vi "ScriptTerminals.vi"(4 "SubVI Refnum":refnum<vi>, 5 "Terms":T1[](array[typedef]), 6 "IS CORE CASE? (f)":bool, 7 "Diag Refnum":refnum<vi>, 9 "error in":errorcluster, 10 "Messages":u8[](array[numeric]), 11 "Name":string) -> ()   [LabVIEW 2012, in "CThread.lvlib"]
uses:
  CThread.lvlib
  <vilib>/XNodeSupport/XNodeTermIDPair.ctl
  <vilib>/XNodeSupport/XNodeTermRef.ctl
  <vilib>/XNodeSupport/XNodeString.ctl
  <vilib>/Utility/miscctls.llb/LVPointTypeDef.ctl
  CRef/CRef.lvlib
  <vilib>/XNodeSupport/NI_XNodeSupport.lvlib
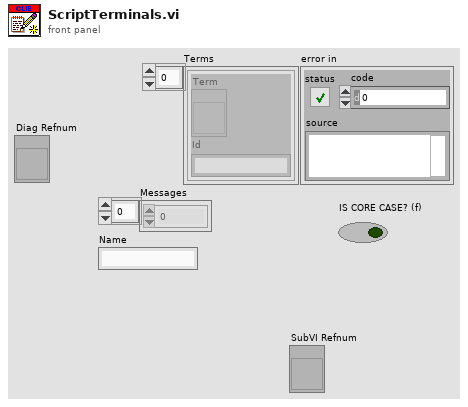
[diagram p1: front panel]
types:
  T1 = typedef "NI_XNodeSupport.lvlib/XNodeTermIDPair.ctl" = cluster{"Term":T2, "Id":T3}
  T2 = typedef "NI_XNodeSupport.lvlib/XNodeTermRef.ctl" = refnum<vi>
  T3 = typedef "NI_XNodeSupport.lvlib/XNodeString.ctl" = string
  T4 = typedef "LVPointTypeDef.ctl" = cluster{"Horizontal":i16, "Vertical":i16}
  T5 = enum16{"Create", "Get", "Set", "Static", "Release"}
  T6 = typedef "CRef.lvlib/Master Types.ctl" = enum8{"Null", "Boolean", "U8", "I8", "U16", "I16", "U32", "I32", "U64", "I64", "Single", "Double", "Extended", "CSG", "CDB", "CXT", "Boolean(Def)", "U8(Def)", "I8(Def)", "U16(Def)", "I16(Def)", "U32(Def)", "I32(Def)", "Reserved Def", "Reserved Def1", "Single(Def)", "Double(Def)", "Reserved Def2", "Reserved Def3", "Reserved Def4", "Reserved Def5", "Unsigned(Def)", "Signed(Def)", "Real(Def)", "Reserved Def6", "Numeric(Def)", "String"}
  T7 = typedef "LVRectTypeDef.ctl" = cluster{"Left":i16, "Top":i16, "Right":i16, "Bottom":i16}
  T8 = cluster{"Left":bool, "Top":bool, "Right":bool, "Bottom":bool}
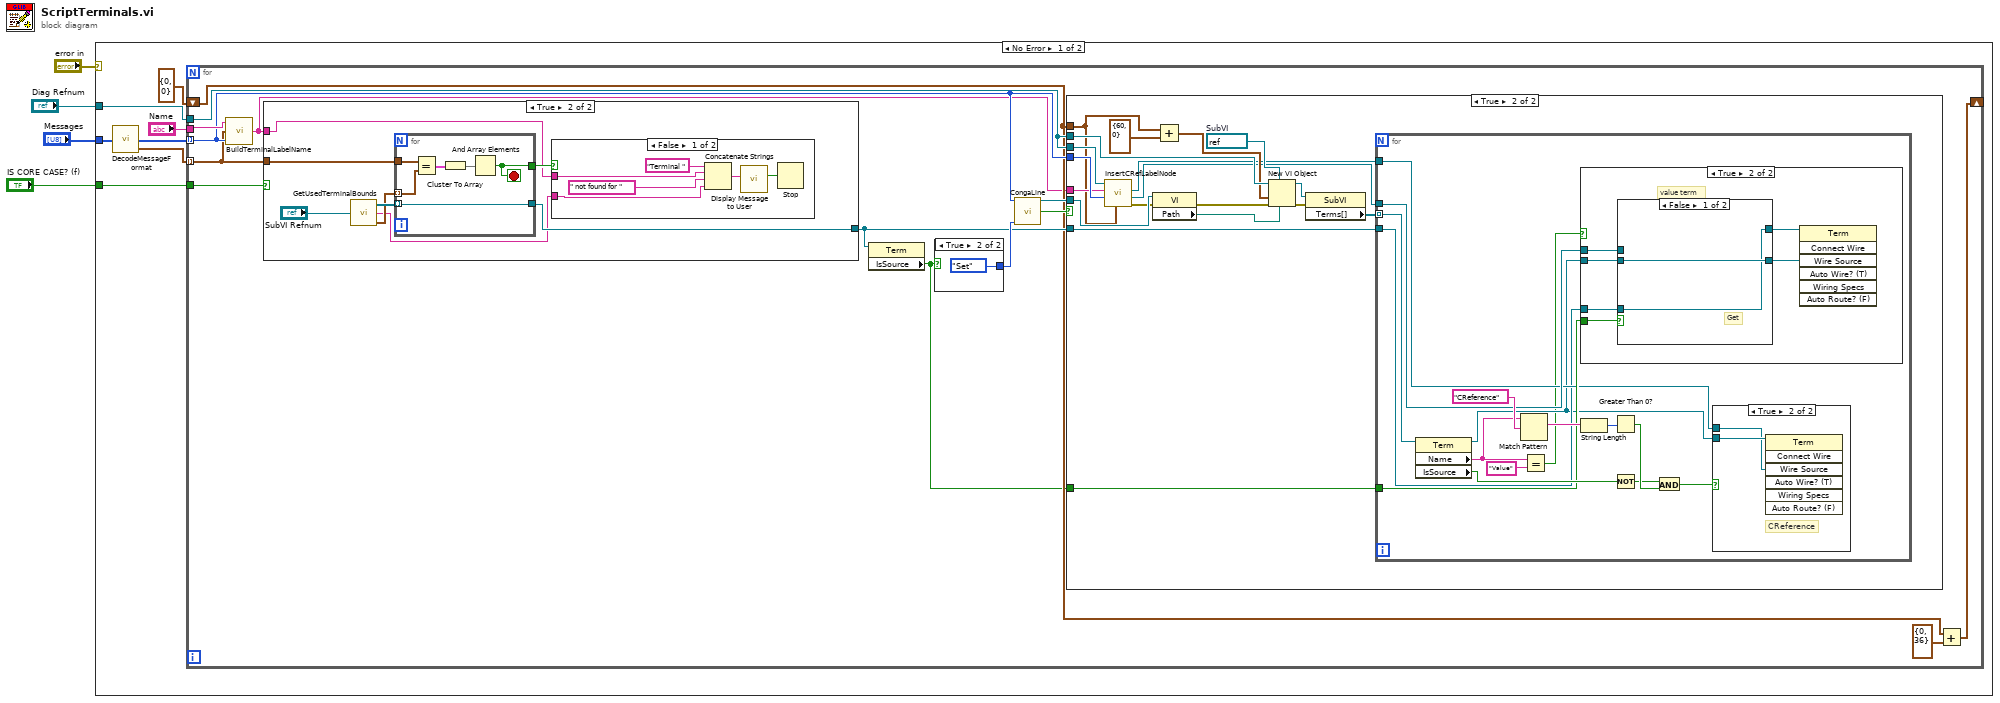
[diagram p0: block diagram]
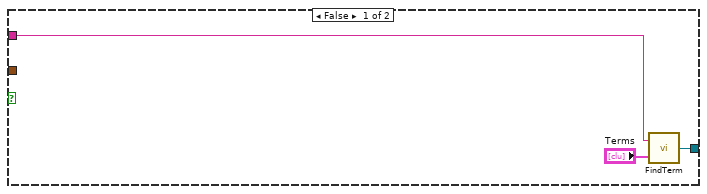
[diagram p2: hidden frame]
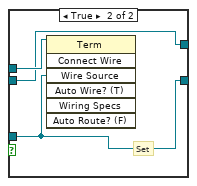
[diagram p6: hidden frame]
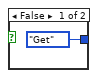
[diagram p8: hidden frame]
diagram:
  n1 = case shown="No Error" "error in" {
    tunnel: "Diag Refnum" -> [w11 _]
    tunnel: "Messages" -> [w5 _]
    tunnel: "IS CORE CASE? (f)" -> [w6 _]
    frame No Error {
      n2 = call "DecodeMessageFormat.vi"("Messages"=w5) -> ("CRef Types"=w10:T6[], "Terminal Bounds[]"=w9:T7[])  [unwired: 2 in, 1 out]
      n3 = for {
        tunnel: w11 -> [w20]
        tunnel: w10 -> [w22] mode=indexing
        tunnel: w9 -> [w13] mode=indexing
        tunnel: "Name" -> [w25]
        shift-right: [w24] -> _
        shift-left: T4 {"Horizontal"=0, "Vertical"=0} ("location") -> [w16]
        tunnel: w6 -> [w14]
        n4 = call "BuildTerminalLabelName.vi"("CRef Type"=w22, "Bounds"=w13, "VI Name"=w25) -> ("Label Name"=w15:string)  [unwired: 1 in]
        n5 = case shown="True" w14 {
          tunnel: [w28 w36] -> w17
          tunnel: w15 -> [w27 w34]
          tunnel: w13 -> [_ w33]
          frame False {
            n6 = call <vilib>:"FindTerm.vi"("Terms"="Terms", "String"=w27) -> ("Term"=w28:refnum<vi>)
          }
          frame True {
            n7 = call "GetUsedTerminalBounds.vi"("SubVI"="SubVI Refnum") -> ("Terminal Bounds[]"=w30:T7[], "VI Name"=w29:string, "Terminals[]"=w31:refnum<vi>[])  [unwired: 2 in]
            n8 = for {
              tunnel: w31 -> [w43] mode=indexing
              tunnel: [w43] -> w36
              tunnel: [w47] -> w35
              tunnel: w33 -> [w45]
              tunnel: w30 -> [w44] mode=indexing
              stop <- w47 stop-if-true
              n9 = Equal?(x=w45, y=w44) -> (x = y?=w46:T8)
              n10 = Cluster To Array(cluster=w46) -> (array=w48:bool[])
              n11 = And Array Elements(Boolean array=w48) -> (logical AND=w47:bool)
            }
            n12 = case shown="False" w35 {
              tunnel: w34 -> [w39 _]
              tunnel: w29 -> [w38 _]
              frame False {
                n13 = Concatenate Strings("Terminal " ("Message"), w39, " not found for " ("Message"), w38) -> (w42:string)
                n14 = call "Display Message to User"("Message"=w42) -> ("OK"=w37:bool)  [unwired: 9 in, 1 out]
                n15 = Stop(stop? (T)=w37) -> ()
              }
              frame True {
              }
            }
          }
        }
        n16 = property class="Term"(reference=w17) -> ("IsSource"=w12:bool)  [unwired: 1 in, 2 out]
        n17 = case shown="True" w12 {
          tunnel: [T5."Get" ("Mode") T5."Set" ("Mode")] -> w21
          frame False {
          }
          frame True {
          }
        }
        n18 = call "CongaLine.vi"("Type"=w22, "Mode"=w21) -> ("vi reference"=w19:refnum<vi>, "implemented?"=w18:bool)  [unwired: 10 in, 2 out]
        n19 = case shown="True" w18 {
          tunnel: w20 -> [_ w67]
          tunnel: w16 -> [_ w55]
          tunnel: w22 -> [_ w66]
          tunnel: w15 -> [_ w65]
          tunnel: w20 -> [_ w64]
          tunnel: w19 -> [_ w62]
          tunnel: w12 -> [_ w52]
          tunnel: w17 -> [_ w49]
          frame False {
          }
          frame True {
            w63 = refnum<vi> refnum  # SubVI
            n20 = call "InsertCRefLabelNode.vi"("location"=w55, "Type"=w66, "Name"=w65, "Diagram"=w67) -> ("error out"=w59:errorcluster, "Init Terminal"=w51:refnum<vi>, "Ref Terminal"=w50:refnum<vi>)  [unwired: 4 in, 1 out]
            n21 = property class="VI"(reference=w62, error in=w59) -> (error out=w60:errorcluster, "Path"=w61:path)  [unwired: 1 out]
            n22 = Add(x=w55, y=T4 {"Horizontal"=60, "Vertical"=0} ("location")) -> (x+y=w53:T4)
            n23 = New VI Object(vi object class=w63, owner refnum=w64, position/next to=w53, 6:w61, 8:w60) -> (object refnum=w57:refnum<vi>, 0:w58:errorcluster)  [unwired: 3 in]
            n24 = property class="SubVI"(reference=w57, error in=w58) -> ("Terms[]"=w56:refnum<vi>[])  [unwired: 2 out]
            n25 = for {
              tunnel: w56 -> [w83] mode=indexing
              tunnel: w52 -> [w76]
              tunnel: w51 -> [w75]
              tunnel: w50 -> [w74]
              tunnel: w49 -> [w71]
              n26 = property class="Term"(reference=w83) -> (reference out=w70:refnum<vi>, "Name"=w68:string, "IsSource"=w78:bool)  [unwired: 1 in, 1 out]
              n27 = Match Pattern(string=w68, regular expression="CReference") -> (match substring=w82:string)  [unwired: 1 in, 3 out]
              n28 = Equal?(x=w68, y="Value" ("regular expression")) -> (x = y?=w69:bool)
              n29 = case shown="True" w69 {
                tunnel: w76 -> [_ w89]
                tunnel: w75 -> [_ w88]
                tunnel: w71 -> [_ w87]
                tunnel: w70 -> [_ w85]
                frame False {
                }
                frame True {
                  # "value term"
                  n30 = case shown="False" w89 {
                    tunnel: w88 -> [_ w94]
                    tunnel: w87 -> [w90 w93]
                    tunnel: [w91 w93] -> w86
                    tunnel: w85 -> [w91 w92]
                    tunnel: [w90 w92] -> w84
                    frame False {
                      # "Get"
                    }
                    frame True {
                      # "Set"
                      n31 = invoke class="Term" method="Connect Wire"(reference=w94, "Wire Source"=w93) -> ()  [unwired: 5 in, 7 out]
                    }
                  }
                  n32 = invoke class="Term" method="Connect Wire"(reference=w84, "Wire Source"=w86) -> ()  [unwired: 5 in, 7 out]
                }
              }
              n33 = String Length(string=w82) -> (length=w81:i32)
              n34 = Greater Than 0?(x=w81) -> (x > 0?=w80:bool)
              n35 = Not(x=w78) -> (.not. x?=w79:bool)
              n36 = And(x=w79, y=w80) -> (x .and. y?=w73:bool)
              n37 = case shown="True" w73 {
                tunnel: w70 -> [_ w96]
                tunnel: w74 -> [_ w95]
                frame False {
                }
                frame True {
                  # "CReference"
                  n38 = invoke class="Term" method="Connect Wire"(reference=w96, "Wire Source"=w95) -> ()  [unwired: 5 in, 7 out]
                }
              }
            }
          }
        }
        n39 = Add(x=w16, y=T4 {"Horizontal"=0, "Vertical"=36}) -> (x+y=w24:T4)
      }
    }
    frame Error {
    }
  }
